vi "find closest match.vi"(4 "start index":i32, 5 "target element":dbl, 6 "tolerance":dbl=inf, 7 "Array":dbl[](array[numeric])) -> (0 "element found?":bool, 1 "element":dbl, 2 "index":i32, 3 "tolerance":dbl)   [LabVIEW 2009]
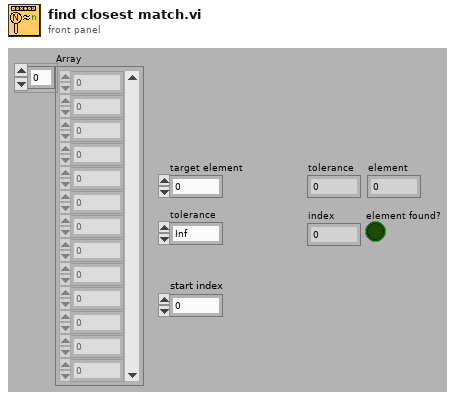
[diagram p1: front panel]
types:
  T1 = cluster{"tolerance":dbl, "index":i32, "element found":dbl}
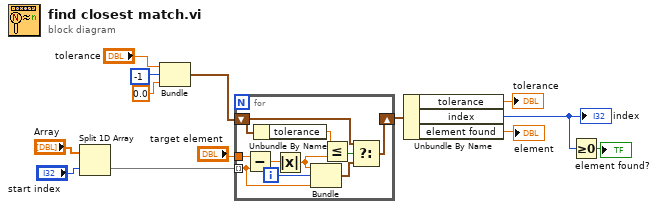
[diagram p0: block diagram]
diagram:
  n1 = Split 1D Array(array="Array", index="start index") -> (second subarray=w1:dbl[])  [unwired: 1 out]
  n2 = Bundle("tolerance"="tolerance", "index"=-1, "element found"=0.0) -> (w9:T1)  [unwired: 1 in]
  n3 = for {
    tunnel: w1 -> [w15] mode=indexing
    tunnel: "target element" -> [w14]
    shift-right: [w18] -> w8
    shift-left: w9 -> [w17]
    i -> [w21]
    n4 = Subtract(x=w14, y=w15) -> (x-y=w23:dbl)
    n5 = Unbundle By Name(w17) -> ("tolerance"=w16:dbl)
    n6 = Absolute Value(x=w23) -> (abs(x)=w19:dbl)
    n7 = Bundle(w19, w21, w15) -> (w20:cluster{dbl, i32, dbl})  [unwired: 1 in]
    n8 = Less Or Equal?(x=w16, y=w19) -> (x <= y?=w22:bool)
    n9 = Select(t=w17, s=w22, f=w20) -> (s? t:f=w18:T1)
  }
  n10 = Unbundle By Name(w8) -> ("tolerance"=→"tolerance":dbl, "index"=w5:i32, "element found"=→"element":dbl)
  "index" <- w5
  n11 = Greater Or Equal To 0?(x=w5) -> (x >= 0?=→"element found?":bool)
